vi "Wheel Speed Sensor.vi"(9 "FPGA I/O In":refnum<k21>="RMC Connector/DIO0") -> (0 "Stopped":bool, 1 "Tick Period":u32, 3 "State Out":bool)   [LabVIEW 2015]
uses:
  <vilib>/rvi/eio/common/nirviEmuTemplateMethod_errors.vi
  <vilib>/eio/EIONode/EIONode.xnode
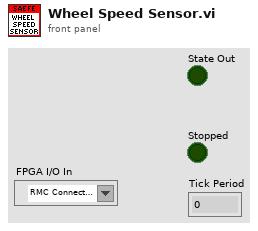
[diagram p1: front panel]
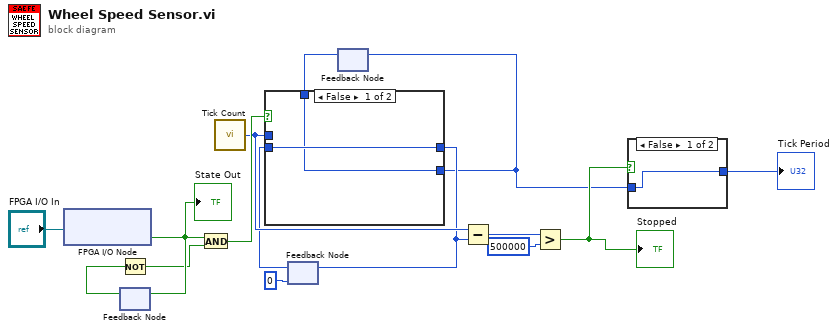
[diagram p0: block diagram]
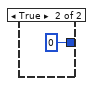
[diagram p2: hidden frame]
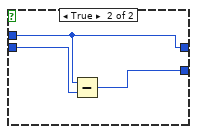
[diagram p3: hidden frame]
diagram:
  n1 = xnode "FPGA I/O Node"("FPGA I/O In"="FPGA I/O In") -> ("I/O Item"=w11:bool)  [unwired: 1 out]
  "State Out" <- w11
  n2 = feedback-in #1(w11) -> ()
  n3 = feedback #1() -> (w10:bool)  [unwired: 1 in]
  n4 = Not(x=w10) -> (.not. x?=w9:bool)
  n5 = And(x=w11, y=w9) -> (x .and. y?=w13:bool)
  n6 = call "Tick Count"() -> ("Tick Count(uSec)"=w8:u32)
  n7 = feedback #2(u32 0 ("Tick Count(uSec)")) -> (w7:u32)
  n8 = feedback #3() -> (w4:u32)  [unwired: 1 in]
  n9 = case shown="False" w13 {
    tunnel: w8 -> [_ w20]
    tunnel: [w17 w20] -> w5
    tunnel: w7 -> [w17 w19]
    tunnel: [w16 w18] -> w2
    tunnel: w4 -> [w16 _]
    frame False {
    }
    frame True {
      n10 = Subtract(x=w20, y=w19) -> (x-y=w18:u32)
    }
  }
  n11 = feedback-in #2(w5) -> ()
  n12 = feedback-in #3(w2) -> ()
  n13 = Subtract(x=w8, y=w5) -> (x-y=w14:u32)
  n14 = Greater?(x=w14, y=u32 500000) -> (0:w3:bool)
  "Stopped" <- w3
  n15 = case shown="False" w3 {
    tunnel: w2 -> [w21 _]
    tunnel: [w21 u32 0] -> w1
    frame False {
    }
    frame True {
    }
  }
  "Tick Period" <- w1
